vi "Example-StaticIO.vi"() -> ()   [LabVIEW 2018]
panel:
  in  "Channel OutEnable":u32=1 format="%.0x"
  in  "Channel OutValue":u32=1 format="%.0x"
  out "布尔数组":bool[](array[boolean])
  in  "停止":bool
  out "returns":i32[](array[numeric])
  out "error out":errorcluster caption="错误输出"
  in  "error in (no error)":errorcluster caption="错误输入（无错误）"
  out "ftHandle out":u64=363562184
  in  "设备索引":i32
  # "1"
  # "4"
  # "8"
  # "12"
  # "16"
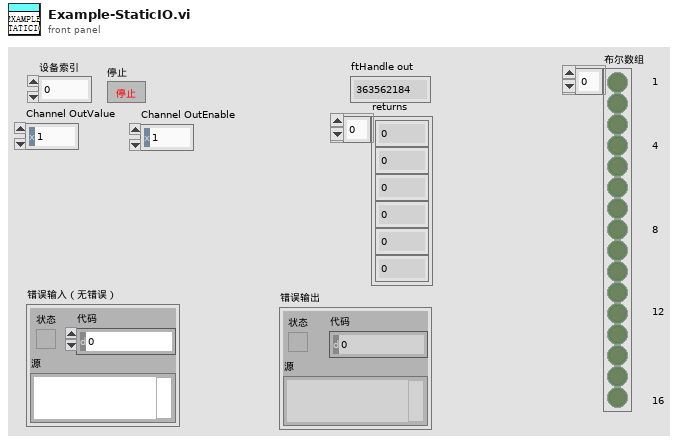
[diagram p1: front panel]
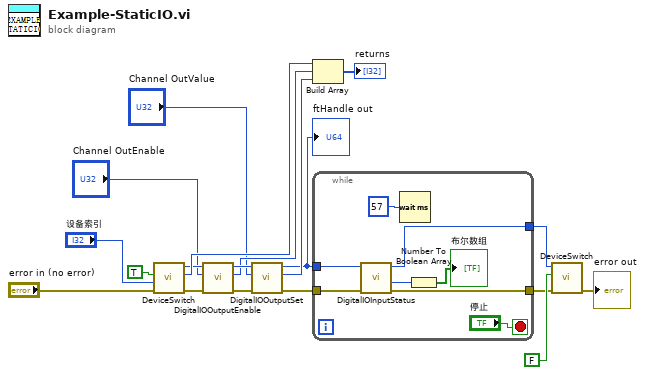
[diagram p0: block diagram]
diagram:
  n1 = call "DeviceSwitch.vi"("error in (no error)"="error in (no error)", "Device Index"="设备索引", "Open"=TRUE) -> ("error out"=w9:errorcluster, "function return"=w15:i32, "handle out"=w10:u64)  [unwired: 4 in, 2 out]
  n2 = call "DigitalIOOutputEnable.vi"("error in (no error)"=w9, "Channel"="Channel OutEnable", "handle"=w10) -> ("error out"=w8:errorcluster, "function return"=w6:i32, "handle out"=w7:u64)  [unwired: 6 in]
  n3 = call "DigitalIOOutputSet.vi"("error in (no error)"=w8, "Channel"="Channel OutValue", "handle"=w7) -> ("error out"=w1:errorcluster, "function return"=w5:i32, "handle out"=w2:u64)  [unwired: 6 in]
  "ftHandle out" <- w2
  n4 = Build Array(w15, w6, w5) -> (→"returns":i32[])
  n5 = while {
    tunnel: w1 -> [w25]
    tunnel: [w24] -> w12
    tunnel: w2 -> [w23]
    tunnel: [w22] -> w11
    stop <- "停止" stop-if-true
    n6 = call "DigitalIOInputStatus.vi"("error in (no error)"=w25, "handle"=w23) -> ("error out"=w24:errorcluster, "reads out"=w21:u32, "handle out"=w22:u64)  [unwired: 6 in, 1 out]
    n7 = Wait (ms)(milliseconds to wait=u32 57 ("等待时间（毫秒）")) -> ()  [unwired: 1 out]
    n8 = Number To Boolean Array(number=w21) -> (Boolean array=→"布尔数组":bool[])
  }
  n9 = call "DeviceSwitch.vi"("error in (no error)"=w12, "Open"=FALSE, "handle"=w11) -> ("error out"=→"error out":errorcluster)  [unwired: 4 in, 4 out]
